vi "Cleanup.vi"(8 "error in (no error)":errorcluster, 11 "Callback Consumer in":refnum<class "Callback Consumer.lvclass">) -> (0 "error out":errorcluster)   [LabVIEW 2012, in "Callback Consumer.lvclass"]
uses:
  Callback Consumer.lvclass
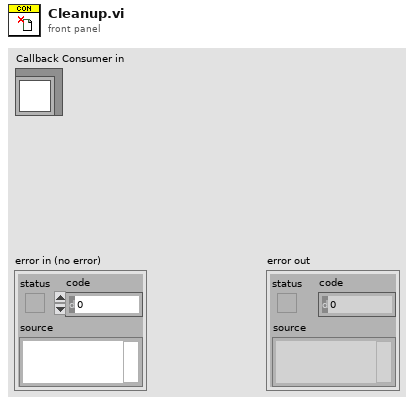
[diagram p1: front panel]
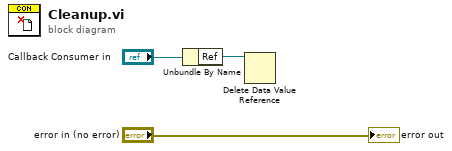
[diagram p0: block diagram]
diagram:
  n1 = Unbundle By Name("Callback Consumer in") -> ("Ref"=w1:refnum<data-value>)
  n2 = Delete Data Value Reference(data value reference=w1) -> ()  [unwired: 1 in, 2 out]
  "error out" <- "error in (no error)"
